vi "Facade.vi"(0 "Data In":T5, 2 "Display State In":T3, 3 "Container State":T4) -> (6 "Data Out":T5, 7 "Display State Out":T3, 8 "Action":T2)   [LabVIEW 2021, in "myRIO MXP.xctl"]
uses:
  <vilib>/myRIO/Common/Instrument Driver Framework/Utilities/xctls/myRIO MXP/myRIO MXP.xctl
  <vilib>/myRIO/Common/Instrument Driver Framework/Utilities/xctls/myRIO MXP/Data.ctl
  <vilib>/_xctls/Container State.ctl
  <vilib>/myRIO/Common/Instrument Driver Framework/Utilities/xctls/myRIO MXP/State.ctl
  <vilib>/_xctls/Action.ctl
  <vilib>/_xctls/XControlSupport.lvlib
panel:
  in  "MXP":T1
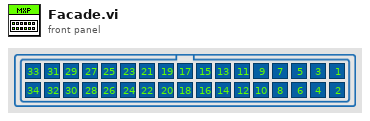
[diagram p1: front panel]
types:
  T1 = cluster{"1":bool, "2":bool, "3":bool, "4":bool, "5":bool, "6":bool, "7":bool, "8":bool, "9":bool, "10":bool, "11":bool, "12":bool, "13":bool, "14":bool, "15":bool, "16":bool, "17":bool, "18":bool, "19":bool, "20":bool, "21":bool, "22":bool, "23":bool, "24":bool, "25":bool, "26":bool, "27":bool, "28":bool, "29":bool, "30":bool, "31":bool, "32":bool, "33":bool, "34":bool}
  T2 = typedef "XControlSupport.lvlib/Action.ctl" = cluster{"Data Changed?":bool, "State Changed?":bool, "Action Name":string}
  T3 = typedef "myRIO MXP.xctl/State.ctl" = cluster{"Pin Disabled?":enum8{"Enabled", "Disabled", "Disabled and Grayed Out"}[], "Pin Name":string[]}
  T4 = typedef "XControlSupport.lvlib/Container State.ctl" = cluster{"Indicator?":bool, "Run Mode?":bool, " Refnum":refnum<vi>}
  T5 = typedef "myRIO MXP.xctl/Data.ctl" = bool[]
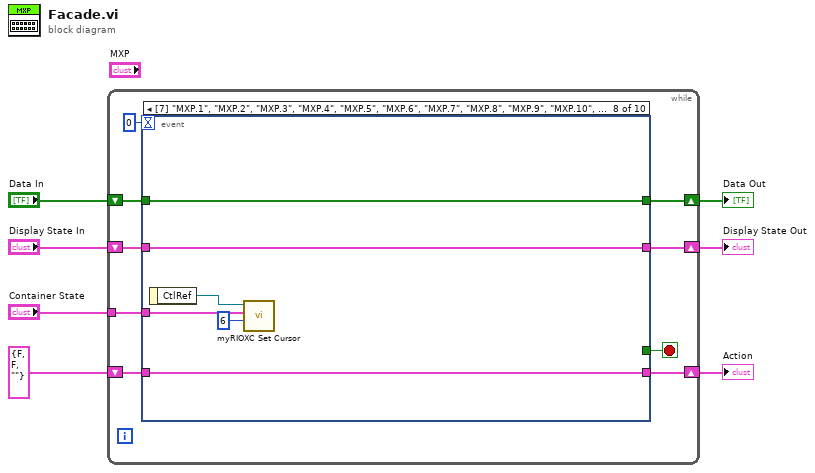
[diagram p0: block diagram]
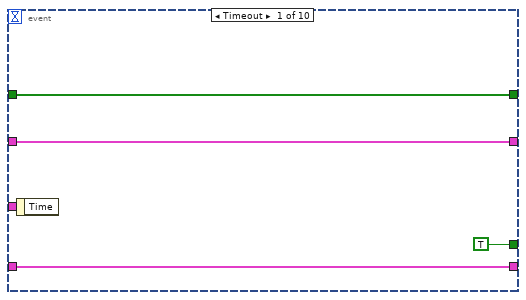
[diagram p2: hidden frame]
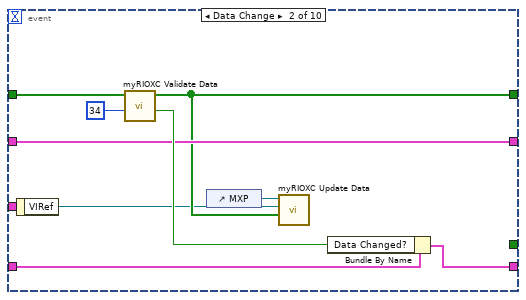
[diagram p3: hidden frame]
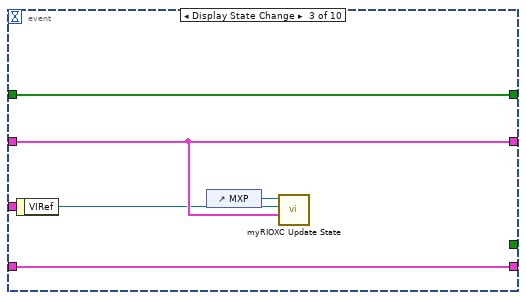
[diagram p4: hidden frame]
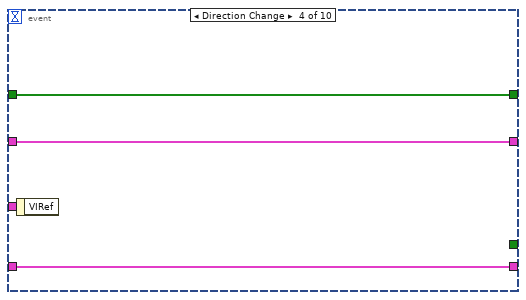
[diagram p5: hidden frame]
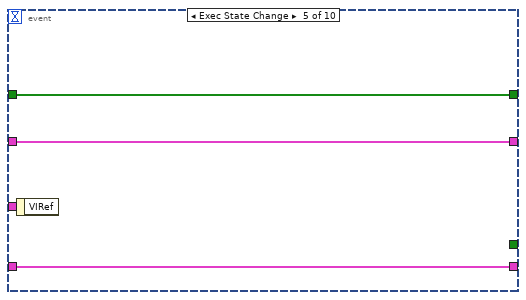
[diagram p6: hidden frame]
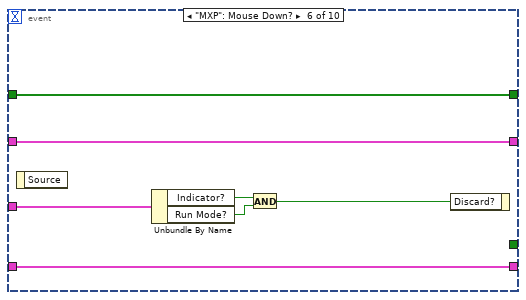
[diagram p7: hidden frame]
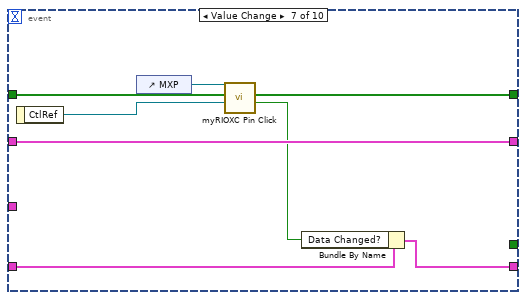
[diagram p8: hidden frame]
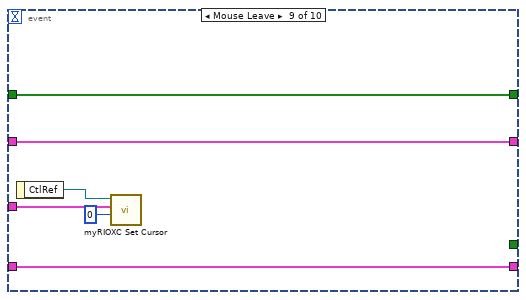
[diagram p9: hidden frame]
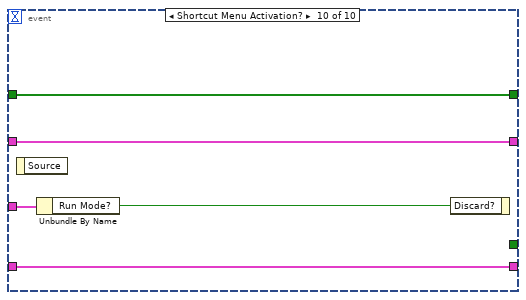
[diagram p10: hidden frame]
diagram:
  n1 = while {
    shift-right: [w16] -> w4
    shift-left: "Display State In" -> [w8]
    tunnel: "Container State" -> [w10]
    shift-right: [w13] -> w7
    shift-left: "Data In" -> [w11]
    shift-right: [w12] -> w2
    shift-left: T2 {"Data Changed?"=FALSE, "State Changed?"=FALSE, "Action Name"=""} ("Action") -> [w9]
    stop <- w15 stop-if-true
    n2 = event shown="[7] \"MXP.1\", \"MXP.2\", \"MXP.3\", \"MXP.4\", \"MXP.5\", \"MXP.6\", \"MXP.7\", \"MXP.8\", \"MXP.9\", \"MXP.10\", \"MXP.11\", \"MXP.12\", \"MXP.13\", \"MXP.14\", \"MXP.15\", \"MXP.16\", \"MXP.17\", \"MXP.18\", \"MXP.19\", \"MXP.20\", \"MXP.21\", \"MXP.22\", \"MXP.23\", \"MXP.24\", \"MXP.25\", \"MXP.26\", \"MXP.27\", \"MXP.28\", \"MXP.29\", \"MXP.30\", \"MXP.31\", \"MXP.32\", \"MXP.33\", \"MXP.34\": Mouse Enter" {
      selector: _ -> [_ _ _ _ _ _ _ _ _ _]
      dyn-events: _ -> [_ _ _ _ _ _ _ _ _ _]
      timeout: 0 -> [_ _ _ _ _ _ _ _ _ _]
      tunnel: w8 -> [w18 w24 w33 w37 w39 w47 w53 w59 w67 w72]
      tunnel: [w18 w24 w33 w37 w39 w47 w53 w59 w67 w72] -> w16
      tunnel: [TRUE _ _ _ _ _ _ _ _ _] -> w15
      tunnel: w10 -> [_ _ _ _ _ w42 _ w56 w62 w69]
      tunnel: w11 -> [w17 w28 w34 w36 w40 w46 w51 w61 w66 w71]
      tunnel: [w17 w23 w34 w36 w40 w46 w50 w61 w66 w71] -> w13
      tunnel: [w19 w26 w32 w35 w38 w45 w54 w60 w65 w70] -> w12
      tunnel: w9 -> [w19 w27 w32 w35 w38 w45 w55 w60 w65 w70]
      event Timeout {
        n3 = event-data() -> ()  [unwired: 1 in, 1 out]
      }
      event Data Change {
        n4 = event-data() -> ("VIRef"=w22:refnum<vi>)  [unwired: 1 in]
        n5 = call <vilib>:"myRIOXC Validate Data.vi"("Size"=34, "Data In"=w28) -> ("Data Changed?"=w25:bool, "Data Out"=w23:bool[])  [unwired: 8 in]
        n6 = control-ref of="MXP"() -> (w21:refnum<vi>)
        n7 = call <vilib>:"myRIOXC Update Data.vi"("Data In"=w23, "Facade Ref"=w22, "Connector Ref"=w21) -> ()  [unwired: 8 in, 1 out]
        n8 = Bundle By Name(cluster=w27, "Data Changed?"=w25) -> (w26:T2)
      }
      event Display State Change {
        n9 = event-data() -> ("VIRef"=w30:refnum<vi>)  [unwired: 1 in]
        n10 = control-ref of="MXP"() -> (w31:refnum<vi>)
        n11 = call <vilib>:"myRIOXC Update State.vi"("Display State In"=w33, "Facade Ref"=w30, "Connector Ref"=w31) -> ()  [unwired: 8 in, 1 out]
      }
      event Direction Change {
        n12 = event-data() -> ()  [unwired: 1 in, 1 out]
      }
      event Exec State Change {
        n13 = event-data() -> ()  [unwired: 1 in, 1 out]
      }
      event "MXP": Mouse Down? {
        n14 = event-data() -> ()  [unwired: 1 in, 1 out]
        n15 = Unbundle By Name(w42) -> ("Indicator?"=w43:bool, "Run Mode?"=w44:bool)
        n16 = And(x=w43, y=w44) -> (x .and. y?=w41:bool)
        n17 = event-data("Discard?"=w41) -> ()  [unwired: 1 in, 1 out]
      }
      event "MXP.1", "MXP.2", "MXP.3", "MXP.4", "MXP.5", "MXP.6", "MXP.7", "MXP.8", "MXP.9", "MXP.10", "MXP.11", "MXP.12", "MXP.13", "MXP.14", "MXP.15", "MXP.16", "MXP.17", "MXP.18", "MXP.19", "MXP.20", "MXP.21", "MXP.22", "MXP.23", "MXP.24", "MXP.25", "MXP.26", "MXP.27", "MXP.28", "MXP.29", "MXP.30", "MXP.31", "MXP.32", "MXP.33", "MXP.34": Value Change {
        # "Value Change"
        n18 = event-data() -> ("CtlRef"=w48:refnum<vi>)  [unwired: 1 in]
        n19 = control-ref of="MXP"() -> (w49:refnum<vi>)
        n20 = call <vilib>:"myRIOXC Pin Click.vi"("Pin Ref"=w48, "Data In"=w51, "Connector Ref"=w49) -> ("Value Change?"=w52:bool, "Data Out"=w50:bool[])  [unwired: 6 in, 1 out]
        n21 = Bundle By Name(cluster=w55, "Data Changed?"=w52) -> (w54:T2)
      }
      event "MXP.1", "MXP.2", "MXP.3", "MXP.4", "MXP.5", "MXP.6", "MXP.7", "MXP.8", "MXP.9", "MXP.10", "MXP.11", "MXP.12", "MXP.13", "MXP.14", "MXP.15", "MXP.16", "MXP.17", "MXP.18", "MXP.19", "MXP.20", "MXP.21", "MXP.22", "MXP.23", "MXP.24", "MXP.25", "MXP.26", "MXP.27", "MXP.28", "MXP.29", "MXP.30", "MXP.31", "MXP.32", "MXP.33", "MXP.34": Mouse Enter {
        n22 = event-data() -> ("CtlRef"=w57:refnum<vi>)  [unwired: 1 in]
        n23 = call <vilib>:"myRIOXC Set Cursor.vi"("Cursor"=u16 6, "Container State"=w56, "PIN Ref"=w57) -> ()  [unwired: 9 in]
      }
      event "MXP.1", "MXP.2", "MXP.3", "MXP.4", "MXP.5", "MXP.6", "MXP.7", "MXP.8", "MXP.9", "MXP.10", "MXP.11", "MXP.12", "MXP.13", "MXP.14", "MXP.15", "MXP.16", "MXP.17", "MXP.18", "MXP.19", "MXP.20", "MXP.21", "MXP.22", "MXP.23", "MXP.24", "MXP.25", "MXP.26", "MXP.27", "MXP.28", "MXP.29", "MXP.30", "MXP.31", "MXP.32", "MXP.33", "MXP.34": Mouse Leave {
        n24 = event-data() -> ("CtlRef"=w63:refnum<vi>)  [unwired: 1 in]
        n25 = call <vilib>:"myRIOXC Set Cursor.vi"("Cursor"=u16 0, "Container State"=w62, "PIN Ref"=w63) -> ()  [unwired: 9 in]
      }
      event Shortcut Menu Activation? {
        n26 = event-data() -> ()  [unwired: 1 in, 1 out]
        n27 = Unbundle By Name(w69) -> ("Run Mode?"=w68:bool)
        n28 = event-data("Discard?"=w68) -> ()  [unwired: 1 in, 1 out]
      }
    }
  }
  "Display State Out" <- w4
  "Data Out" <- w7
  "Action" <- w2
